vi "ForTmpTest.vi"() -> ()   [LabVIEW 2014]
uses:
  <vilib>/Instr/_visa.llb/VISA Configure Serial Port (Instr).vi
panel:
  out "read buffer":string
  out "ERRIn?":string
  in  "VISA resource name":refnum<visa-resource-name>
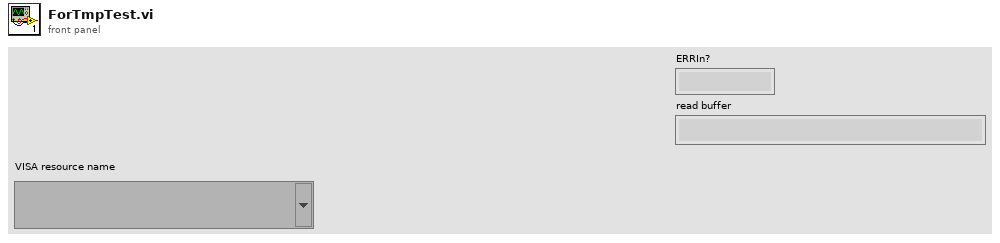
[diagram p1: front panel]
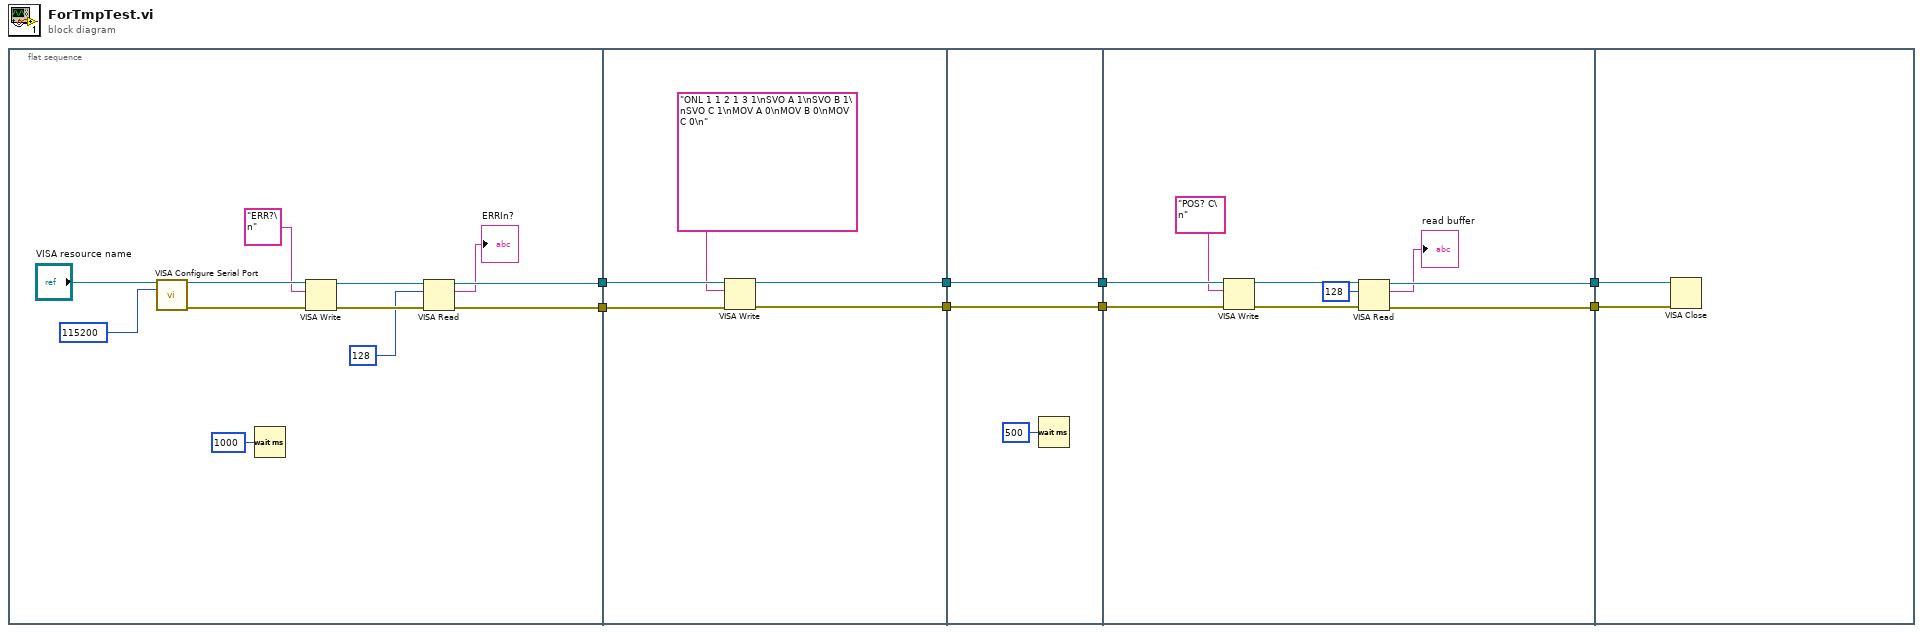
[diagram p0: block diagram]
diagram:
  n1 = flat-sequence {
    tunnel: [w12] -> w8
    tunnel: [w11] -> w7
    tunnel: w8 -> [w25]
    tunnel: w7 -> [w24]
    tunnel: [w22] -> w6
    tunnel: [w21] -> w5
    tunnel: w6 -> [w28]
    tunnel: [w28] -> w4
    tunnel: w5 -> [w27]
    tunnel: [w27] -> w2
    tunnel: w4 -> [w37]
    tunnel: [w33] -> w3
    tunnel: w2 -> [w36]
    tunnel: [w32] -> w1
    tunnel: w3 -> [w39]
    tunnel: w1 -> [w38]
    frame #0 {
      n2 = call-poly "VISA Configure Serial Port"("VISA resource name"="VISA resource name", "baud rate (9600)"=u32 115200) -> ("VISA resource name out"=w17:refnum<visa-resource-name>, "error out"=w16:errorcluster)  [unwired: 12 in]
      n3 = Wait (ms)(milliseconds to wait=u32 1000) -> ()  [unwired: 1 out]
      n4 = VISA Write(VISA resource name=w17, write buffer="ERR?\n", error in (no error)=w16) -> (VISA resource name out=w14:refnum<visa-resource-name>, error out=w13:errorcluster)  [unwired: 1 out]
      n5 = VISA Read(VISA resource name=w14, byte count=u32 128, error in (no error)=w13) -> (VISA resource name out=w12:refnum<visa-resource-name>, read buffer=→"ERRIn?":string, error out=w11:errorcluster)  [unwired: 1 out]
    }
    frame #1 {
      n6 = VISA Write(VISA resource name=w25, write buffer="ONL 1 1 2 1 3 1\nSVO A 1\nSVO B 1\nSVO C 1\nMOV A 0\nMOV B 0\nMOV C 0\n", error in (no error)=w24) -> (VISA resource name out=w22:refnum<visa-resource-name>, error out=w21:errorcluster)  [unwired: 1 out]
    }
    frame #2 {
      n7 = Wait (ms)(milliseconds to wait=u32 500) -> ()  [unwired: 1 out]
    }
    frame #3 {
      n8 = VISA Write(VISA resource name=w37, write buffer="POS? C\n", error in (no error)=w36) -> (VISA resource name out=w35:refnum<visa-resource-name>, error out=w34:errorcluster)  [unwired: 1 out]
      n9 = VISA Read(VISA resource name=w35, byte count=u32 128, error in (no error)=w34) -> (VISA resource name out=w33:refnum<visa-resource-name>, read buffer=→"read buffer":string, error out=w32:errorcluster)  [unwired: 1 out]
    }
    frame #4 {
      n10 = VISA Close(VISA resource name=w39, error in (no error)=w38) -> ()  [unwired: 1 out]
    }
  }
